vi "Get Self Queue.vi"(11 "Model_AMC in":refnum<class "Model_AMC.lvclass">) -> (3 "Self queue":T1)   [LabVIEW 2021, in "Model_AMC.lvclass"]
uses:
  Model_AMC.lvclass
  <userlib>/John_Lib/AMC_FW/AMC_SelfCustom/Queue.ctl
  <userlib>/John_Lib/AMC_FW/Message Queue.ctl
  <userlib>/John_Lib/AMC_FW/Message.ctl
  <userlib>/John_Lib/AMC_FW/Tools/Keyed Array/KeyedArray.ctl
  Model_AMC.lvclass/Model_AMC.ctl
  <userlib>/John_Lib/AMC_FW/Tools/Keyed Array/Tools_KeyedArray.lvlib
  <userlib>/John_Lib/AMC_FW/AMC_FW.lvlib
panel:
  out "error out":errorcluster
  in  "error in (no error)":errorcluster
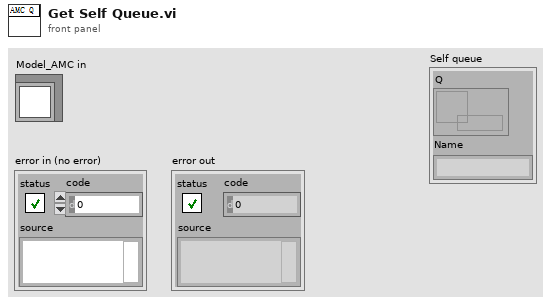
[diagram p1: front panel]
types:
  T1 = typedef "AMC_FW.lvlib/Queue.ctl" = cluster{"Q":T2, "Name":string}
  T2 = typedef "AMC_FW.lvlib/Message Queue.ctl" = refnum<queue>
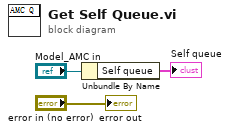
[diagram p0: block diagram]
diagram:
  n1 = Unbundle By Name("Model_AMC in") -> ("Self queue"=→"Self queue":T1)
  "error out" <- "error in (no error)"
